vi "Write MeasurementsToRead.vi"(8 "error in (no error)":errorcluster, 10 "MeasurementsToRead":T1=[{"Type"="Internal Temp F", "OID"="1.3.6.1.4.1.20916.1.6.1.1.1.1.0"}, {"Type"="Internal Temp C", "OID"="1.3.6.1.4.1.20916.1.6.1.1.1.2.0"}, {"Type"="Digital Sensor 1 Temp C", "OID"="1.3.6.1.4.1.20916.1.6.1.2.1.1.0"}, {"Type"="Digital Sensor 1 Temp F", "OID"="1.3.6.1.4.1.20916.1.6.1.2.1.2.0"}, {"Type"="Digital Sensor 2 Temp C", "OID"="1.3.6.1.4.1.20916.1.6.1.2.2.1.0"}, {"Type"="Digital Sensor 2 Temp F", "OID"="1.3.6.1.4.1.20916.1.6.1.2.2.2.0"}, {"Type"="Switch Sensor State", "OID"="1.3.6.1.4.1.20916.1.6.1.3.1.0"}, {"Type"="Signal Tower Red State", "OID"="1.3.6.1.4.1.20916.1.6.2.1.0"}, {"Type"="Signal Tower Amber State", "OID"="1.3.6.1.4.1.20916.1.6.2.2.0"}, {"Type"="Signal Tower Green State", "OID"="1.3.6.1.4.1.20916.1.6.2.3.0"}, {"Type"="Signal Tower Alarm 1", "OID"="1.3.6.1.4.1.20916.1.6.2.6.0"}, {"Type"="Alarm Message", "OID"="1.3.6.1.4.1.20916.1.6.3.1.0"}], 11 "RoomAlert in":refnum<class "RoomAlert.lvclass">) -> (0 "error out":errorcluster, 3 "RoomAlert out":refnum<class "RoomAlert.lvclass">)   [LabVIEW 2018, in "SensorPlugins.lvlib" / "RoomAlert.lvclass"]
uses:
  RoomAlert.lvclass
  TypeDefinitions/MeasurementToRead.ctl
  RoomAlert.lvclass/RoomAlert.ctl
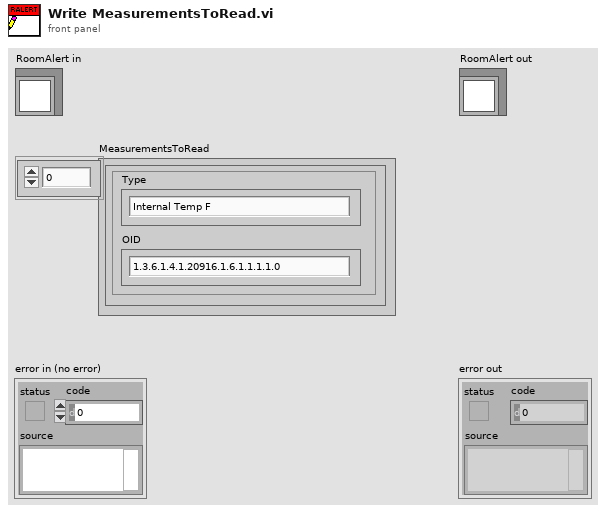
[diagram p1: front panel]
types:
  T1 = typedef "SensorPlugins.lvlib/RoomAlert.lvclass/MeasurementToRead.ctl" = cluster{"Type":string, "OID":string}[]
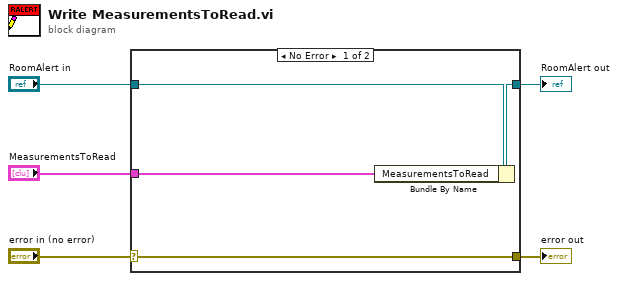
[diagram p0: block diagram]
diagram:
  n1 = case shown="No Error" "error in (no error)" {
    selector: "error in (no error)" -> [w9 w10]
    tunnel: [w9 w10] -> w4
    tunnel: [w7 w11] -> w2
    tunnel: "RoomAlert in" -> [w8 w11]
    tunnel: "MeasurementsToRead" -> [w6 _]
    frame No Error {
      n2 = Bundle By Name(cluster=w8, "MeasurementsToRead"=w6) -> (w7:refnum<class "RoomAlert.lvclass">)
    }
    frame Error {
    }
  }
  "error out" <- w4
  "RoomAlert out" <- w2
